vi "Get Client Python File.vi"() -> (3 "appended path":path)   [LabVIEW 2025]
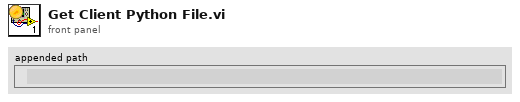
[diagram p1: front panel]
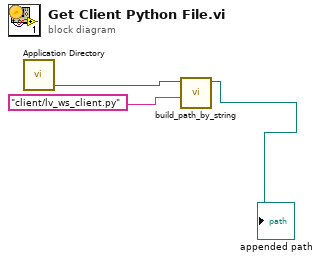
[diagram p0: block diagram]
diagram:
  n1 = call <vilib>:"Application Directory.vi"() -> ("Application Directory"=w2:path)
  n2 = call "build_path_by_string.vi"("String"="client/lv_ws_client.py", "base path"=w2) -> ("appended path"=→"appended path":path)  [unwired: 9 in]
